vi "Async RTL Read Test.vi"() -> ()   [LabVIEW 2016]
panel:
  out "LVUserEventRef":refnum<user-event>
  out "BufferLength":u32
  out "NumberOfBuffers":u32
  out "return type":i32
  out "Sample Rate (Hz)":u32
  out "Data":i8[](array[numeric])
  out "Boolean":bool
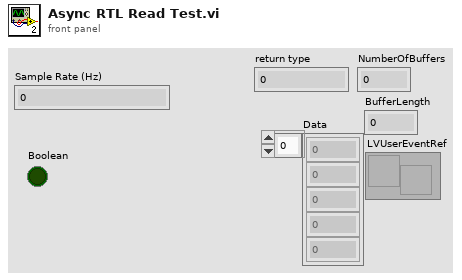
[diagram p1: front panel]
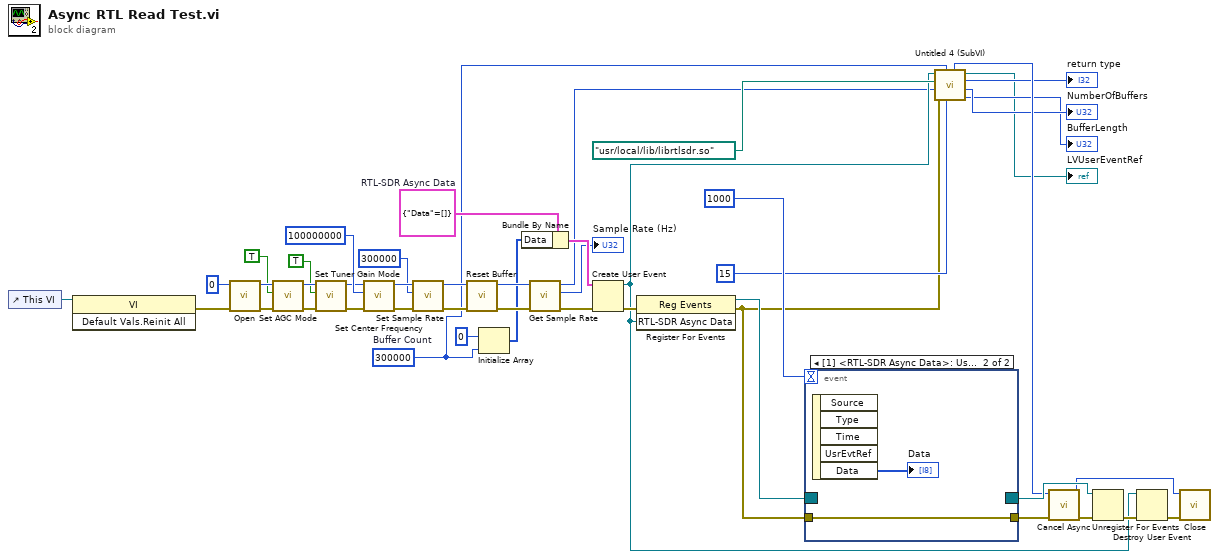
[diagram p0: block diagram]
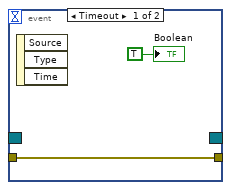
[diagram p2: hidden frame]
diagram:
  w10 = 300000  # Buffer Count
  w28 = cluster{"Data":i8[]} {"Data"=[]}  # RTL-SDR Async Data
  n1 = control-ref of="This VI"() -> (w18:refnum<vi>)
  n2 = invoke class="VI" method="Default Vals.Reinit All"(reference=w18) -> (error out=w17:errorcluster)  [unwired: 2 in, 2 out]
  n3 = call "Open.vi"("error in (no error)"=w17, "Device Index"=u32 0) -> ("error out"=w34:errorcluster, "DeviceRefnum Out"=w36:u64)  [unwired: 6 in]
  n4 = call "Set AGC Mode.vi"("error in (no error)"=w34, "AGC Enable"=TRUE, "DeviceRefnum"=w36) -> ("error out"=w33:errorcluster, "DeviceRefnum Out"=w35:u64)  [unwired: 6 in, 1 out]
  n5 = call "Set Tuner Gain Mode.vi"("error in (no error)"=w33, "AutoGain"=TRUE, "DeviceRefnum"=w35) -> ("error out"=w31:errorcluster, "DeviceRefnum Out"=w32:u64)  [unwired: 6 in, 1 out]
  n6 = call "Set Center Frequency.vi"("error in (no error)"=w31, "Center Frequency"=u32 100000000, "DeviceRefnum"=w32) -> ("error out"=w40:errorcluster, "DeviceRefnum Out"=w41:u64)  [unwired: 6 in, 1 out]
  n7 = call "Set Sample Rate.vi"("error in (no error)"=w40, "Sample Rate"=u32 300000, "DeviceRefnum"=w41) -> ("error out"=w38:errorcluster, "DeviceRefnum Out"=w39:u64)  [unwired: 6 in, 1 out]
  n8 = call "Reset Buffer.vi"("error in (no error)"=w38, "DeviceRefnum"=w39) -> ("error out"=w24:errorcluster, "DeviceRefnum Out"=w22:u64)  [unwired: 7 in, 1 out]
  n9 = Initialize Array(i8 0, w10) -> (w19:i8[])
  n10 = Bundle By Name(cluster=w28, "Data"=w19) -> (w27:cluster{"Data":i8[]})
  n11 = call "Get Sample Rate.vi"("error in (no error)"=w24, "DeviceRefnum"=w22) -> ("error out"=w23:errorcluster, "Sample Rate (Hz)"=→"Sample Rate (Hz)":u32, "DeviceRefnum Out"=w7:u64)  [unwired: 7 in]
  n12 = Create User Event(user event datatype=w27, error in=w23) -> (user event=w13:refnum<user-event>, error out=w16:errorcluster)
  n13 = register-events(error in=w16, w13) -> (reference out=w26:refnum<event-registration>, error out=w11:errorcluster)  [unwired: 1 in]
  n14 = event shown="[1] <RTL-SDR Async Data>: User Event" {
    selector: w26 -> [_ _]
    dyn-events: [_ _] -> w25
    timeout: 1000 -> [_ _]
    tunnel: [w46 w49] -> w9
    tunnel: w11 -> [w46 w49]
    event Timeout {
      n15 = event-data() -> ()  [unwired: 1 in, 3 out]
      "Boolean" <- TRUE ("Boolean")
    }
    event User Event {
      n16 = event-data() -> ("Data"=→"Data":i8[])  [unwired: 1 in, 4 out]
    }
  }
  n17 = call "Untitled 4 (SubVI).vi"("NumberOfBuffers in"=u32 15 ("NumberOfBuffers"), "Buffer Count"=w10, "error in (no error)"=w11, "DeviceRefnum In"=w7, "path in"=path "/usr/local/lib/librtlsdr.so", "User Event in"=w13) -> ("BufferLength"=→"BufferLength":u32, "NumberOfBuffers out"=→"NumberOfBuffers":u32, "return type"=→"return type":i32, "User Event out"=→"LVUserEventRef":refnum<user-event>, "DeviceRefnum Out"=w6:u64)  [unwired: 1 in]
  n18 = call "Cancel Async.vi"("error in (no error)"=w9, "DeviceRefnum"=w6) -> ("error out"=w8:errorcluster, "DeviceRefnum Out"=w5:u64)  [unwired: 7 in]
  n19 = Unregister For Events(event registration refnum=w25, error in=w8) -> (error out=w42:errorcluster)
  n20 = Destroy User Event(user event=w13, error in=w42) -> (error out=w15:errorcluster)
  n21 = call "Close.vi"("error in (no error)"=w15, "DeviceRefnum"=w5) -> ()  [unwired: 8 in, 2 out]
